vi "Icai 105 - Simultry2.vi"() -> ()   [LabVIEW 2010]
uses:
  <vilib>/Utility/error.llb/DialogType.ctl
  <vilib>/DAQmx/write.llb/DAQmx Write (Analog DBL 1Chan 1Samp).vi
  <vilib>/DAQmx/write.llb/DAQmx Write (Analog Wfm 1Chan NSamp).vi
  <vilib>/DAQmx/create/channels.llb/DAQmx Create Channel (AO-Voltage-Basic).vi
  <vilib>/daqmx/miscellaneous.llb/DAQmx Fill In Error Info.vi
  <vilib>/Waveform/WDTOps.llb/WDT Append Waveforms DBL.vi
  <vilib>/measure/NI_MABase.lvlib
  Program Files/National Instruments/LabVIEW 2010/resource/objmgr/daqmx.rc
panel:
  in  "Modulation Duration samples / 2":i32=150000
  out "Multiplier to arrive at Modulation # of samples":dbl=297.555285
  in  "Samples (1Ms/s)":i32=1000000
  out "Name":refnum<k21>
  out "number of samples written per channel":u32
  out "max value":dbl
  in  "Logic Output Channel":tag="Dev1/ao3"
  in  "FM Waveform Channel":tag="Dev1/ao2"
  out "error out":errorcluster caption="error out (DAQ)"
  out "Mod":dbl=118572.0
  out "Numeric 2":dbl=3900000.0 format="%#_7g"
  out "Numeric":dbl=3900000.0 format="%#_7g"
  in  "CAI/ICAI":bool=TRUE
  in  "Pre-Trig Samples":ext=1140.74 format="%.2f"
  out "?":dbl=579698.7113293351 format="%#_6f"
  in  "Fs":dbl=1000000.0
  out "#s":dbl=39524.02451426849
  in  "Time int":i32=30000
  in  "Sensitivity":u16(ring)=14 items=["2 nV/fA", "5 nV/fA", "10 nV/fA", "20 nV/fA", "50 nV/fA", "100 nV/fA", "200 nV/fA", "500 nV/fA", "1 uV/pA", "2 uV/pA", "5 uV/pA", "10 uV/pA", "20 uV/pA", "50 uV/pA", "100 uV/pA", "200 uV/pA", "500 uV/pA", "1 mV/nA", "2 mV/nA", "5 mV/nA", "10 mV/nA", "20 mV/nA", "50 mV/nA", "100 mV/nA", "200 mV/nA", "500 mV/nA", "1 V/uA"]
  in  "Detection Bandwidth":u16(ring)=7 items=["25 kHz", "8.33 kHz", "2.50 kHz", "833 Hz", "250 Hz", "83.3 Hz", "25 Hz", "8.33 Hz", "2.50 Hz", "0.833 Hz", "0.250 Hz", "0.0833 Hz", "0.025 Hz"]
  in  "SR 830 GPIB Address":i32=8
  in  "Freq 2":dbl=897.8 format="%_7g"
  out "Iterat #":dbl=10.0
  in  "Iteration":dbl=2.0
  in  "stop 2":bool
  in  "pulse":bool=TRUE
  in  "Start":ext=0.05
  out "?":waveform(dbl)[](graph)=[{"t0"=timestamp(0 s since 1904-01-01), "dt"=1e-06, "Y"=array[3900000 elements]}, {"t0"=timestamp(0 s since 1904-01-01), "dt"=1e-06, "Y"=array[3900000 elements]}]
  in  "amplitude 2":dbl=1.0 format="%0.2p"
  in  "?":T1(ring)
  in  "phase 2":dbl format="%.2p"
  in  "Offset 2":dbl=-0.0 format="%#_6p"
  in  "frequency 4":dbl=100.0 format="%0.2p"
  in  "sampling info 4":cluster{"Fs":dbl, "#s":dbl}={"Fs"=1000000.0, "#s"=2500.0} {"Fs" format="%.2p"}
  in  "?":T1(ring)=enum."Triangle Wave"
  in  "offset 4":dbl=-1.0 format="%0.2p"
  in  "phase 4":dbl=90.0 format="%.2p"
  in  "amplitude 4":dbl=1.0 format="%0.2p"
  in  "frequency 1":dbl=100.0 format="%0.2p"
  in  "amplitude 1":dbl=1.0 format="%0.2p"
  in  "sampling info 1":cluster{"Fs":dbl, "#s":dbl}={"Fs"=1000000.0, "#s"=2500.0} {"Fs" format="%.2p"}
  in  "?":T1(ring)=enum."Triangle Wave"
  in  "phase 1":dbl=-90.0 format="%.2p"
  in  "Offset 1":dbl format="%#_6p"
  in  "iterat":dbl=1.0
  out "CW":dbl=123571.0
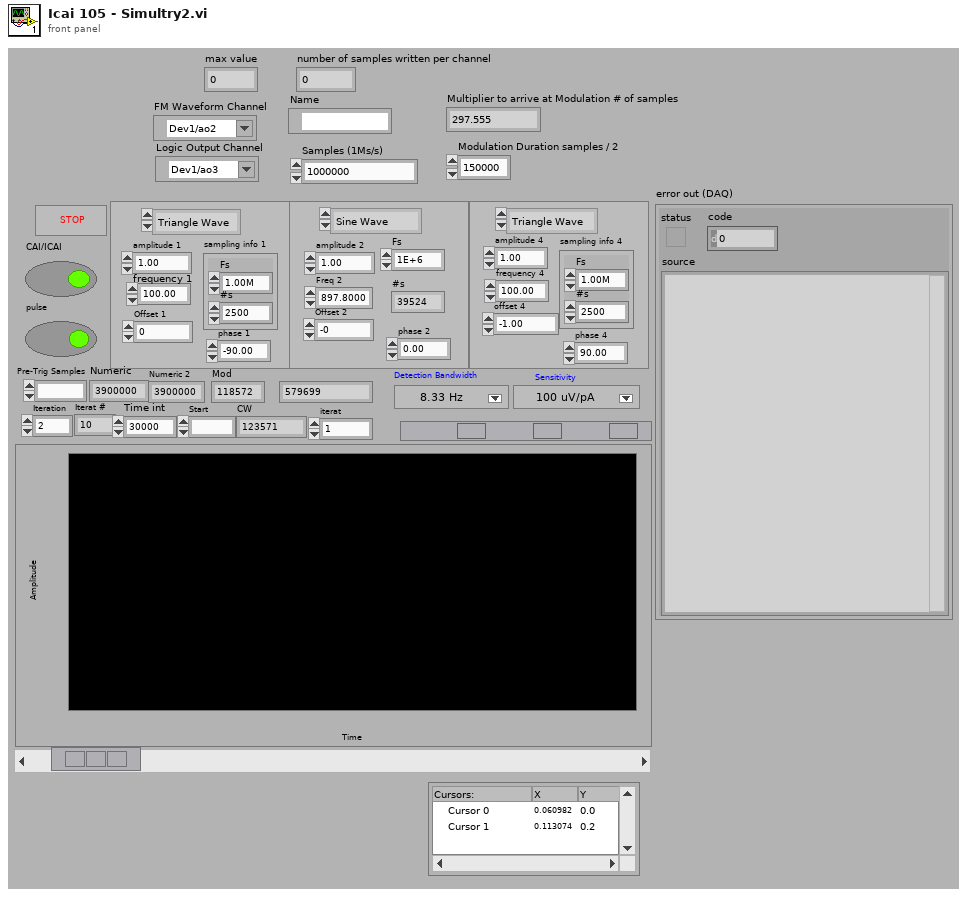
[diagram p1: front panel]
types:
  T1 = enum16{"Sine Wave", "Triangle Wave", "Square Wave", "Sawtooth Wave"}
  T2 = typedef "DialogType.ctl" = u16
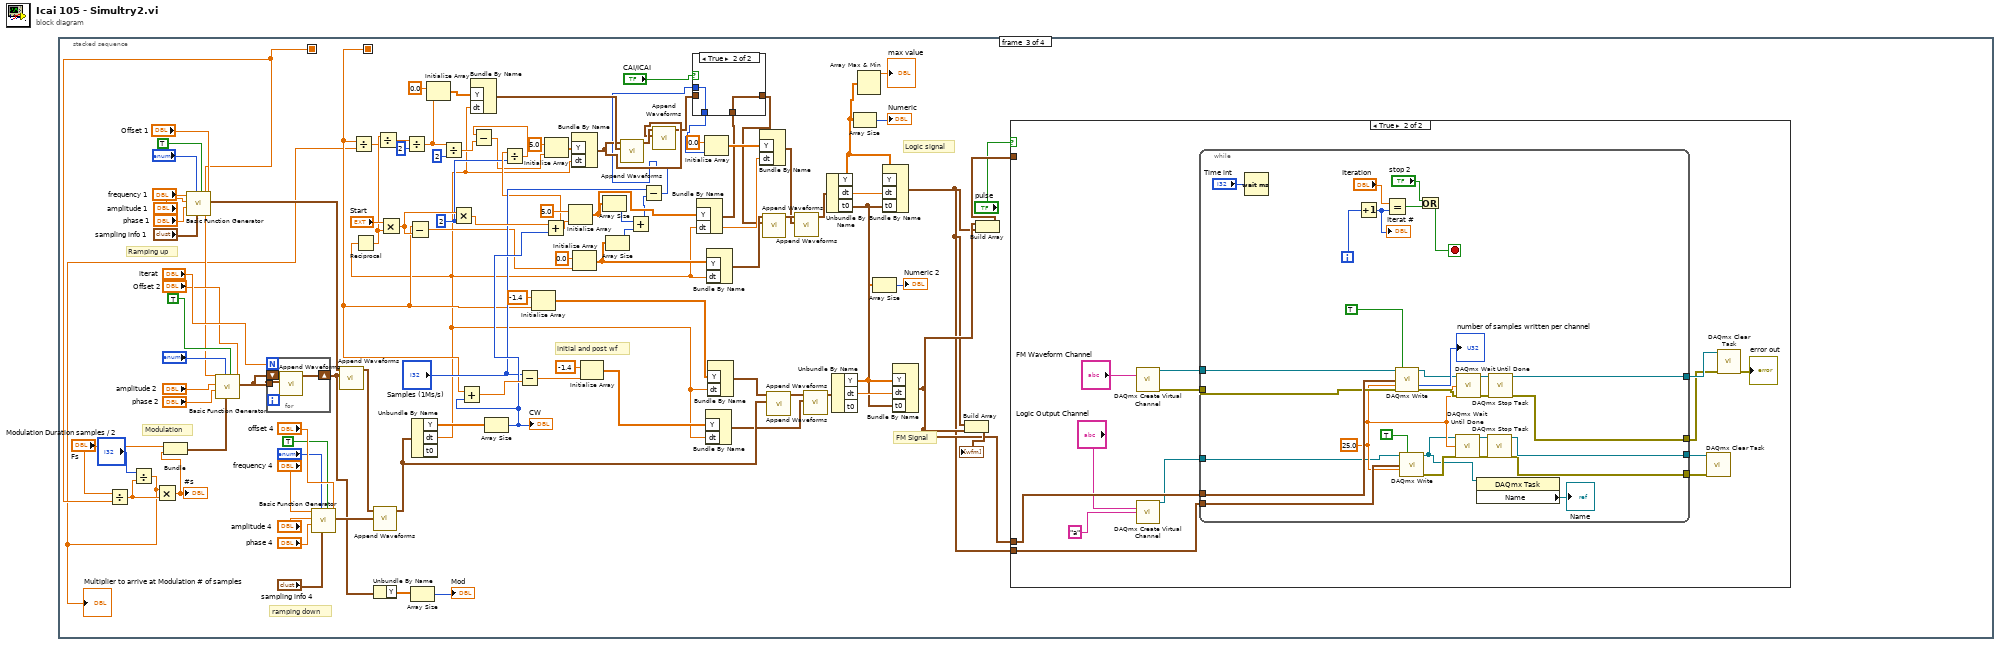
[diagram p0: block diagram]
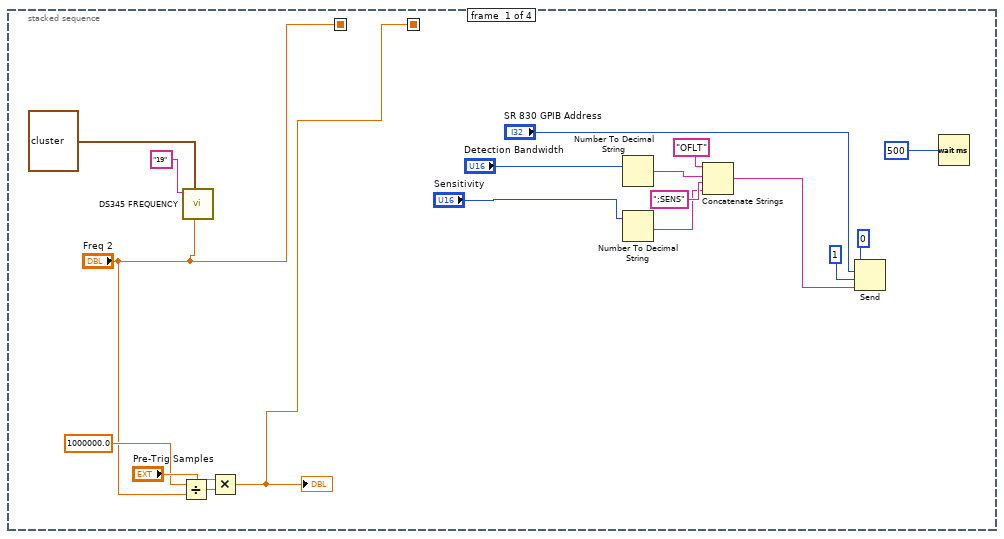
[diagram p2: hidden frame]
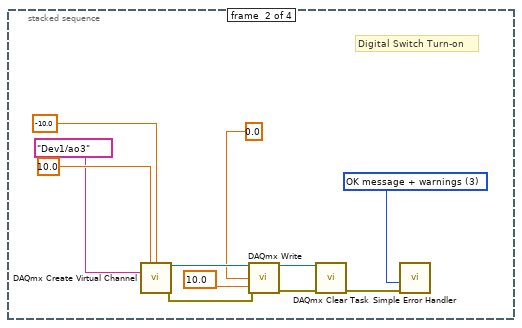
[diagram p3: hidden frame]
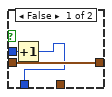
[diagram p4: hidden frame]
diagram:
  n1 = stacked-sequence {
    seq-local: ["Freq 2" _ _ _] -> [_ _ w72 _]
    seq-local: [w2 _ _ _] -> [_ _ w59 _]
    frame #0 {
      n2 = Divide(x=1000000.0 ("Fs 2"), y="Freq 2") -> (x/y=w5:dbl)
      n3 = call "DS345 FREQUENCY.vi"("GPIB address"="19", "amplitude (0 Vrms:0)"=cluster{ext, i32} {0.02, 0} ("Driving amplitude (0 Vrms:0)"), "frequency"="Freq 2") -> ()  [unwired: 5 in, 1 out]
      n4 = Multiply(x="Pre-Trig Samples", y=w5) -> (x*y=w2:ext)
      "?" <- w2
      n5 = Number To Decimal String(number="Detection Bandwidth") -> (decimal integer string=w15:string)  [unwired: 1 out]
      n6 = Number To Decimal String(number="Sensitivity") -> (decimal integer string=w13:string)  [unwired: 1 out]
      n7 = Concatenate Strings("OFLT", w15, ";SENS", w13) -> (w12:string)
      n8 = Send(0:0 ("bus"), 2:"SR 830 GPIB Address", 3:i16 1 ("mode"), 5:w12) -> ()  [unwired: 1 in, 3 out]
      n9 = Wait (ms)(milliseconds to wait=500) -> ()  [unwired: 1 out]
    }
    frame #1 {
      w22 = T2 3 items=["no dialog", "OK message", "continue or stop message", "OK message + warnings", "continue/stop + warnings"] ("type of dialog (OK msg:1)")
      # "Digital Switch Turn-on"
      n10 = call-poly <vilib>:"DAQmx Create Virtual Channel.vi"("maximum value"=10.0 ("Maximum Value"), "minimum value"=-10.0 ("Minimum Value"), "physical channels"=tag "Dev1/ao3" ("Physical Channel")) -> ("task out"=w25:refnum<k21>, "error out"=w26:errorcluster)  [unwired: 6 in, 5 out]
      n11 = call-poly <vilib>:"DAQmx Write.vi"("task/channels in"=w25, "data"=0.0 ("Voltage Output"), "timeout"=10.0, "error in"=w26) -> ("task out"=w20:refnum<k21>, "error out"=w21:errorcluster)  [unwired: 1 in, 9 out]
      n12 = call <vilib>:"DAQmx Clear Task.vi"("task in"=w20, "error in"=w21) -> ("error out"=w19:errorcluster)  [unwired: 13 out]
      n13 = call <vilib>:"Simple Error Handler.vi"("type of dialog (OK msg:1)"=w22, "error in (no error)"=w19) -> ()  [unwired: 8 out]
    }
    frame #2 {
      w67 = 2
      # "initial and post wf"
      # "FM Signal"
      # "Logic signal"
      # "Ramping up"
      # "ramping down"
      # "Modulation"
      n14 = Divide(x="Fs", y=w72) -> (x/y=w31:dbl)
      n15 = Divide(x="Modulation Duration samples / 2", y=w31) -> (x/y=w30:dbl)
      "Multiplier to arrive at Modulation # of samples" <- w30
      n16 = Multiply(x=w30, y=w31) -> (x*y=w33:dbl)
      "#s" <- w33
      n17 = Bundle("Fs"="Fs", w33) -> (w70:cluster{"Fs":dbl, dbl})  [unwired: 1 out]
      n18 = call <vilib>:"Basic Function Generator.vi"("offset"="Offset 1", "reset signal"=TRUE, "sampling info"="sampling info 1", "signal type"="?", "phase"="phase 1", "amplitude"="amplitude 1", "frequency"="frequency 1") -> ("signal out"=w112:waveform(dbl))  [unwired: 2 in, 2 out]
      n19 = call <vilib>:"Basic Function Generator.vi"("offset"="Offset 2", "reset signal"=TRUE, "sampling info"=w70, "signal type"="?", "phase"="phase 2", "amplitude"="amplitude 2", "frequency"=w72) -> ("signal out"=w73:waveform(dbl))  [unwired: 2 in, 2 out]
      n20 = for {
        N: "iterat" -> [_]
        shift-right: [w183] -> w38
        shift-left: w73 -> [w181]
        tunnel: w73 -> [w182]
        n21 = call-poly <vilib>:"Append Waveforms.vi"("waveform B"=w182, "waveform A"=w181) -> ("waveform out"=w183:waveform(dbl))  [unwired: 1 in, 8 out]
      }
      n22 = call <vilib>:"Basic Function Generator.vi"("offset"="offset 4", "reset signal"=TRUE, "sampling info"="sampling info 4", "signal type"="?", "phase"="phase 4", "amplitude"="amplitude 4", "frequency"="frequency 4") -> ("signal out"=w117:waveform(dbl))  [unwired: 2 in, 2 out]
      n23 = call-poly <vilib>:"Append Waveforms.vi"("waveform B"=w38, "waveform A"=w112) -> ("waveform out"=w111:waveform(dbl))  [unwired: 1 in, 8 out]
      n24 = Divide(x=w59, y=w30) -> (x/y=w60:ext)
      n25 = call-poly <vilib>:"Append Waveforms.vi"("waveform B"=w117, "waveform A"=w111) -> ("waveform out"=w110:waveform(dbl))  [unwired: 1 in, 8 out]
      n26 = Unbundle By Name(w38) -> ("Y"=w39:dbl[])
      n27 = Array Size(array=w39) -> (size(s)=→"Mod":i32)
      n28 = Unbundle By Name(w110) -> ("Y"=w113:dbl[], "dt"=w51:dbl)  [unwired: 1 out]
      n29 = Reciprocal(x=w51) -> (1/x=w61:dbl)
      n30 = Divide(x=w61, y=w60) -> (x/y=w57:ext)
      n31 = Multiply(x="Start", y=w61) -> (x*y=w84:ext)
      n32 = Divide(x=w57, y=2) -> (x/y=w54:ext)
      n33 = Subtract(x=w59, y=w84) -> (x-y=w85:ext)
      n34 = Initialize Array(0.0 ("Trigger down"), w54) -> (w64:dbl[])
      n35 = Divide(x=w54, y=2) -> (x/y=w52:ext)
      n36 = Multiply(x=w84, y=w67) -> (x*y=w92:ext)
      n37 = Bundle By Name("Y"=w64, "dt"=w51) -> (w63:waveform(dbl))  [unwired: 1 out]
      n38 = Array Size(array=w113) -> (size(s)=w91:i32)
      "CW" <- w91
      n39 = Add(x=w59, y=w91) -> (x+y=w96:ext)
      n40 = Subtract(x="Samples (1Ms/s)", y=w96) -> (x-y=w95:ext)
      n41 = Initialize Array(-1.4 ("DC level"), w59) -> (w98:dbl[])
      n42 = Add(x=w92, y=w91) -> (x+y=w68:ext)
      n43 = Divide(x=w68, y=w67) -> (x/y=w56:ext)
      n44 = Subtract(x=w56, y=w52) -> (x-y=w55:ext)
      n45 = Initialize Array(5.0 ("Trigger up"), w55) -> (w66:dbl[])
      n46 = Initialize Array(5.0 ("Trigger up"), w68) -> (w82:dbl[])
      n47 = Bundle By Name("Y"=w66, "dt"=w51) -> (w50:waveform(dbl))  [unwired: 1 out]
      n48 = Initialize Array(0.0 ("Trigger down"), w85) -> (w83:dbl[])
      n49 = Initialize Array(-1.4 ("DC level"), w95) -> (w94:dbl[])
      n50 = Array Size(array=w82) -> (size(s)=w80:i32)
      n51 = Array Size(array=w83) -> (size(s)=w81:i32)
      n52 = call-poly <vilib>:"Append Waveforms.vi"("waveform B"=w63, "waveform A"=w50) -> ("waveform out"=w62:waveform(dbl))  [unwired: 1 in, 8 out]
      n53 = Add(x=w80, y=w81) -> (x+y=w79:i32)
      n54 = Subtract(x="Samples (1Ms/s)", y=w79) -> (x-y=w42:i32)
      n55 = call-poly <vilib>:"Append Waveforms.vi"("waveform B"=w50, "waveform A"=w62) -> ("waveform out"=w49:waveform(dbl))  [unwired: 1 in, 8 out]
      n56 = Bundle By Name("Y"=w82, "dt"=w51) -> (w47:waveform(dbl))  [unwired: 1 out]
      n57 = case shown="True" "CAI/ICAI" {
        tunnel: w49 -> [w136 _]
        tunnel: [w136 w138] -> w48
        tunnel: w47 -> [_ w138]
        tunnel: w42 -> [w135 w137]
        tunnel: [w134 w137] -> w41
        frame False {
          n58 = Increment(x=w135) -> (x+1=w134:i32)
        }
        frame True {
        }
      }
      n59 = Initialize Array(0.0 ("Trigger down"), w41) -> (w88:dbl[])
      n60 = Bundle By Name("Y"=w94, "dt"=w51) -> (w93:waveform(dbl))  [unwired: 1 out]
      n61 = Bundle By Name("Y"=w83, "dt"=w51) -> (w87:waveform(dbl))  [unwired: 1 out]
      n62 = Bundle By Name("Y"=w98, "dt"=w51) -> (w115:waveform(dbl))  [unwired: 1 out]
      n63 = Bundle By Name("Y"=w88, "dt"=w51) -> (w86:waveform(dbl))  [unwired: 1 out]
      n64 = call-poly <vilib>:"Append Waveforms.vi"("waveform B"=w48, "waveform A"=w87) -> ("waveform out"=w107:waveform(dbl))  [unwired: 1 in, 8 out]
      n65 = call-poly <vilib>:"Append Waveforms.vi"("waveform B"=w110, "waveform A"=w115) -> ("waveform out"=w116:waveform(dbl))  [unwired: 1 in, 8 out]
      n66 = call-poly <vilib>:"Append Waveforms.vi"("waveform B"=w86, "waveform A"=w107) -> ("waveform out"=w103:waveform(dbl))  [unwired: 1 in, 8 out]
      n67 = call-poly <vilib>:"Append Waveforms.vi"("waveform B"=w93, "waveform A"=w116) -> ("waveform out"=w101:waveform(dbl))  [unwired: 1 in, 8 out]
      n68 = Unbundle By Name(w103) -> ("Y"=w37:dbl[], "dt"=w102:dbl, "t0"=w78:timestamp)
      n69 = Unbundle By Name(w101) -> ("Y"=w43:dbl[], "dt"=w100:dbl)  [unwired: 1 out]
      n70 = Array Size(array=w37) -> (size(s)=→"Numeric":i32)
      n71 = Array Max & Min(array=w37) -> (max value=→"max value":dbl)  [unwired: 3 out]
      n72 = Array Size(array=w43) -> (size(s)=→"Numeric 2":i32)
      n73 = Bundle By Name("Y"=w37, "dt"=w102, "t0"=w78) -> (w34:waveform(dbl))  [unwired: 1 out]
      n74 = Bundle By Name("Y"=w43, "dt"=w100, "t0"=w78) -> (w35:waveform(dbl))  [unwired: 1 out]
      n75 = Build Array(w34, w35) -> (→"?":waveform(dbl)[])
      n76 = Build Array(w35, w34) -> (w104:waveform(dbl)[])
      n77 = case shown="True" "pulse" {
        tunnel: w104 -> [_ _]
        tunnel: w35 -> [_ w151]
        tunnel: w34 -> [_ w147]
        frame False {
        }
        frame True {
          n78 = call-poly <vilib>:"DAQmx Create Virtual Channel.vi"("physical channels"="FM Waveform Channel") -> ("task out"=w149:refnum<k21>, "error out"=w148:errorcluster)  [unwired: 13 in]
          n79 = call-poly <vilib>:"DAQmx Create Virtual Channel.vi"("physical channels"="Logic Output Channel", "name to assign"="a") -> ("task out"=w145:refnum<k21>)  [unwired: 12 in, 1 out]
          n80 = while {
            tunnel: w151 -> [w167]
            tunnel: w149 -> [w161]
            tunnel: w148 -> [w160]
            tunnel: w147 -> [w164]
            tunnel: w145 -> [w158]
            tunnel: [w155] -> w143
            tunnel: [w154] -> w142
            tunnel: [w153] -> w141
            tunnel: [w152] -> w140
            i -> [w177]
            stop <- w178 stop-if-true
            w159 = 25.0 ("timeout (s)")
            n81 = Wait (ms)(milliseconds to wait="Time int") -> ()  [unwired: 1 out]
            n82 = Increment(x=w177) -> (x+1=w175:i32)
            "Iterat #" <- w175
            n83 = Equal?(x="Iteration", y=w175) -> (x = y?=w180:bool)
            n84 = call-poly <vilib>:"DAQmx Write.vi"("task/channels in"=w161, "auto start"=TRUE, "data"=w167, "timeout"=w159, "error in"=w160) -> ("task out"=w169:refnum<k21>, "number of samples written per channel"=→"number of samples written per channel":u32, "error out"=w168:errorcluster)  [unwired: 8 in]
            n85 = call-poly <vilib>:"DAQmx Write.vi"("task/channels in"=w158, "auto start"=TRUE, "data"=w164, "timeout"=w159) -> ("task out"=w157:refnum<k21>, "error out"=w165:errorcluster)  [unwired: 9 in, 1 out]
            n86 = Or(x="stop 2", y=w180) -> (x .or. y?=w178:bool)
            n87 = call <vilib>:"DAQmx Wait Until Done.vi"("task/channels in"=w157, "timeout (sec)"=w159, "error in"=w165) -> ("task out"=w163:refnum<k21>, "error out"=w166:errorcluster)  [unwired: 11 in]
            n88 = call <vilib>:"DAQmx Wait Until Done.vi"("task/channels in"=w169, "timeout (sec)"=w159, "error in"=w168) -> ("task out"=w173:refnum<k21>, "error out"=w172:errorcluster)  [unwired: 11 in]
            n89 = property class="DAQmx Task"(reference=w157) -> ("Name"=→"Name":refnum<k21>)  [unwired: 1 in, 2 out]
            n90 = call <vilib>:"DAQmx Stop Task.vi"("task/channels in"=w163, "error in"=w166) -> ("task out"=w155:refnum<k21>, "error out"=w154:errorcluster)  [unwired: 12 in]
            n91 = call <vilib>:"DAQmx Stop Task.vi"("task/channels in"=w173, "error in"=w172) -> ("task out"=w153:refnum<k21>, "error out"=w152:errorcluster)  [unwired: 12 in]
          }
          n92 = call <vilib>:"DAQmx Clear Task.vi"("task in"=w143, "error in"=w142) -> ()  [unwired: 13 in, 1 out]
          n93 = call <vilib>:"DAQmx Clear Task.vi"("task in"=w141, "error in"=w140) -> ("error out"=→"error out":errorcluster)  [unwired: 13 in]
        }
      }
    }
    frame #3 {
    }
  }
